vi "lowpass.vi"(1 "Tau_P-1":i16, 2 "In":i16) -> (0 "Out":i16)   [LabVIEW 2010, in "Wall Follower.lvrbt"]
uses:
  Wall Follower.lvrbt
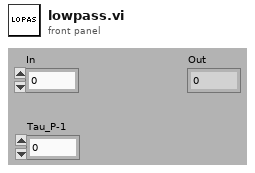
[diagram p1: front panel]
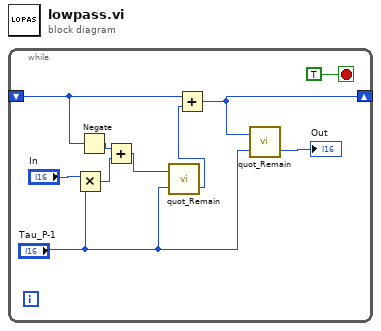
[diagram p0: block diagram]
diagram:
  n1 = while {
    shift-right: [w3] -> _
    shift-left: _ -> [w8]
    stop <- TRUE stop-if-true
    n2 = Multiply(x="In", y="Tau_P-1") -> (x*y=w4:i16)
    n3 = Negate(x=w8) -> (-x=w9:i32)
    n4 = Add(x=w9, y=w4) -> (x+y=w7:i32)
    n5 = call <vilib>:"quot_Remain.vi"("y"="Tau_P-1", "x"=w7) -> ("floor(x/y)"=w6:i32)  [unwired: 1 out]
    n6 = Add(x=w8, y=w6) -> (x+y=w3:i32)
    n7 = call <vilib>:"quot_Remain.vi"("y"="Tau_P-1", "x"=w3) -> ("floor(x/y)"=→"Out":i32)  [unwired: 1 out]
  }
